vi "GUI_Cameras_v1.3.1.vi"() -> ()   [LabVIEW 2013]
uses:
  <vilib>/vision/NI_Vision_Development_Module.lvlib
  <vilib>/Utility/miscctls.llb/LVRectTypeDef.ctl
panel:
  in  "resize":bool
  in  "Tab Control":T1(tab)
  out "Max Counts":dbl(slide) scale=0.0..256.0
  in  "triggerdelay":dbl
  in  "trigger":bool
  in  "save":bool
  in  "exposure":dbl=0.52 caption="Exposure"
  in  "gain":dbl
  in  "shotnumber":i32=354
  in  "LogArray":bool
  in  "ROI.OffsetY":dbl
  in  "ROI.OffsetX":dbl
  in  "ROI.Height":dbl
  in  "ROI.Width":dbl
  in  "localanalysis":bool
  in  "MaxGUIPixel":dbl
  out "Centroid":cluster{"X Centroid":sgl, "Y Centroid":sgl} {"Y Centroid" format="%.2f"; "X Centroid" format="%.2f"}
  out "Y Resolution":i32
  out "X Resolution":i32
  out "Mean Value":sgl format="%.2f"
  out "GUIBinning":dbl
  in  "size":dbl=20.0
  in  "Target.Y":dbl
  in  "Target.X":dbl
  in  "draw Xhair":bool
  out "Mean Value 2":sgl(graph)
  out "histogram":T2(graph)
  out "lineout":cluster{"x0":sgl, "dx":sgl, "Pixels Line":sgl[]}(graph)
  out "MaxCounts":dbl
  in  "FWHMx":dbl
  in  "FWHMy":dbl
  out "MeanCounts":dbl
  out "FWHMx (um)":dbl
  out "FWHMy (um)":dbl
  in  "SpatialCalibration":dbl
  in  "Analysis":bool
  out "analysis error":errorcluster
  out "top":i16
  out "left":i16
  out "Zoom changed":bool
  out "Zoom old":cluster{"X":sgl, "Y":sgl}
  out "ratio(h)":bool=TRUE
  out "fixsize":bool
  out "Change Ratio":cluster{"X":sgl, "Y":sgl}={"X"=1.6671598, "Y"=0.6151203}
  out "old Panel Bounds":T3={"Left"=105, "Top"=80, "Right"=781, "Bottom"=662}
  out "error (h)":bool
  in  "Main Tap":enum32{"IMAQ", "Network", "Internal", "Array"}(tab)
  out "Image (IMAQ)":T4(plugin-control)
  out "local Port":u16=65401
  out "Remote Host":string="192.168.10.157"
  out "port or service name":u16=65400
  in  "timeout ms (slow resp)":i32=500
  in  "reset":bool
  out "All Devices (h)":string[](array[string])
  out "centroidy":dbl
  out "fast ID (h)":refnum<k16>
  out "slow ID (h)":refnum<k16>
  out "error out":errorcluster
  out "connections (hidden)":variant[](array[variant])=[variant(refnum<k16> refnum), variant(refnum<k16> refnum)]
  in  "time to wait (main loop)":i32=200
  in  "time to wait (TCP)":i32=10
  out "Data String":string="exposure,0.520000\r\ntrigger,off\r\nsave,off\r\ngain,0.000000\r\n"
  in  "send":bool
  in  "localsavingpath":path
  out "centroidy":dbl
  out "Image (array)":dbl[][](graph)
  out "Device Name (h)":string="FakeCam1"
  out "stop":bool
  out "error message":string
  out "image connection":bool
  out "data connection ok":bool
  # "Trigger"
  # "Save"
  # "Data"
  # "Image"
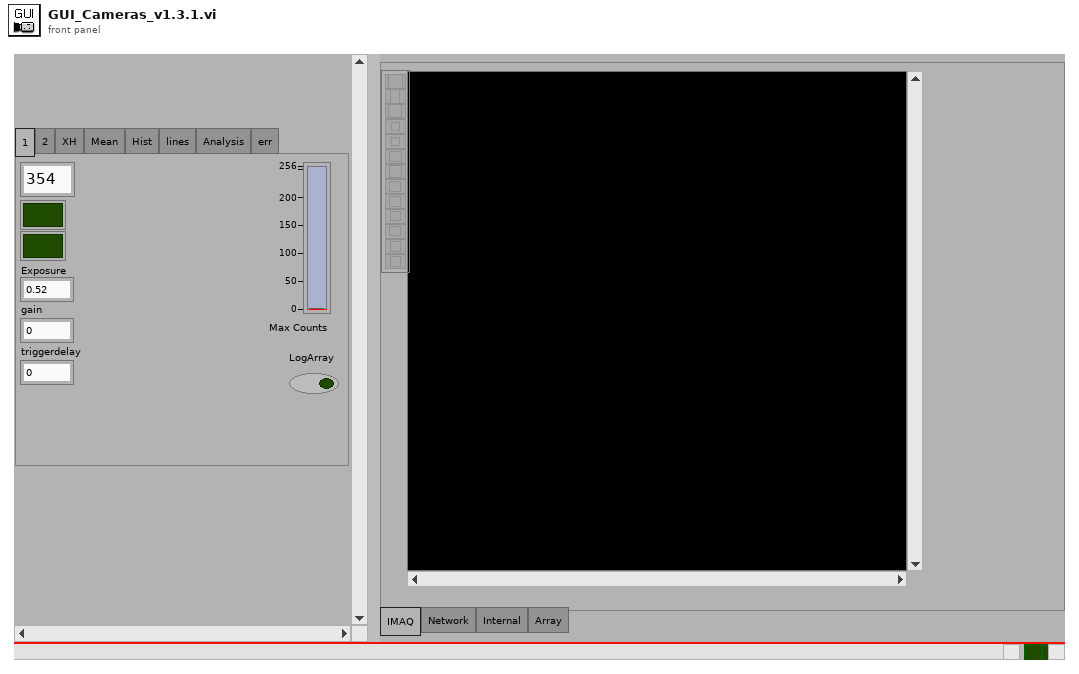
[diagram p1: front panel]
types:
  T1 = enum32{"1", "2", "XH", "Mean", "Hist", "lines", "Analysis", "err"}
  T2 = cluster{"Starting Value":sgl, "Incremental Value":sgl, "Histogram":u32[]}
  T3 = typedef "LVRectTypeDef.ctl" = cluster{"Left":i16, "Top":i16, "Right":i16, "Bottom":i16}
  T4 = typedef "IMAQ Image.ctl" = refnum<image>
  T5 = enum16{"Grayscale", "Binary", "Gradient", "Rainbow", "Temperature", "User Defined"}
  T6 = cluster{"Left":i32, "Top":i32, "Right":i32, "Bottom":i32}
  T7 = typedef "Image Type" = u32
  T8 = cluster{"Global Rectangle":i32[], "Contours":cluster{"Contour Type":u32, "ROI Type":u32, "Points":i32[]}[]}
  T9 = typedef "EventTypDef.ctl" = refnum<user-event>
  T10 = typedef "IMAQ Line" = cluster{"Start X":i32, "Start Y":i32, "End X":i32, "End Y":i32}
  T11 = typedef "LVBoundsTypeDef.ctl" = cluster{"Width":u32, "Height":u32}
  T12 = typedef "ROI Descriptor" = cluster{"Global Rectangle":i32[], "Contours":cluster{"ID":enum32{"External", "Internal"}, "Type":u32, "Coordinates":i32[]}[]}
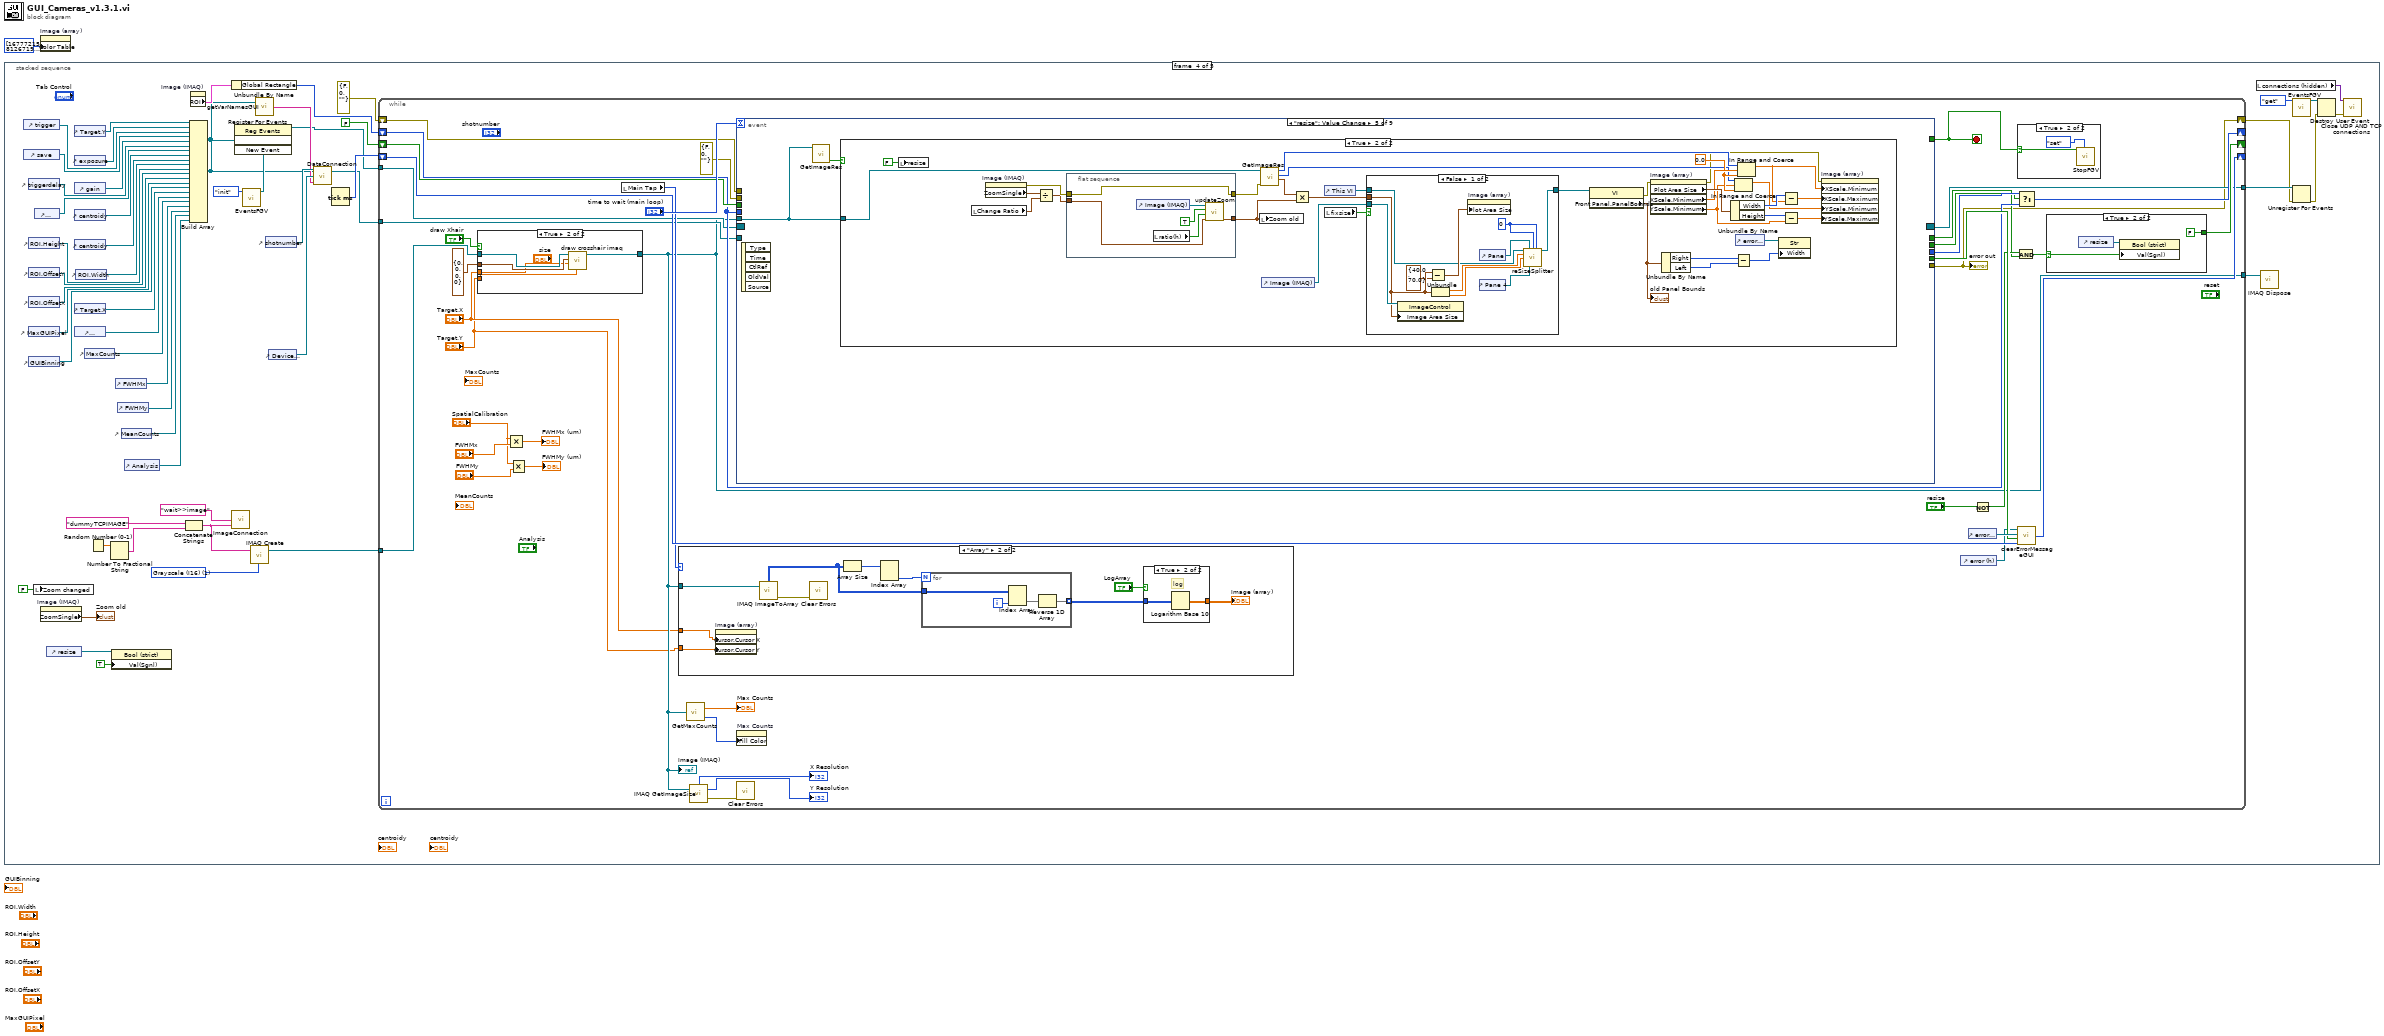
[diagram p0: block diagram]
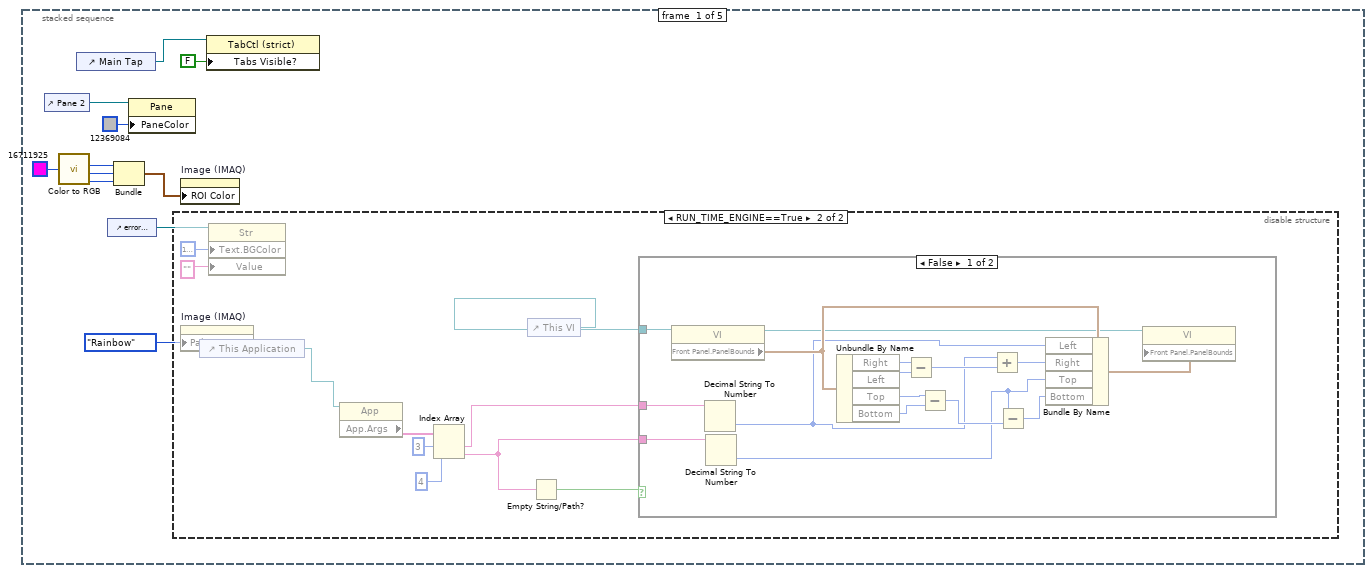
[diagram p2: hidden frame]
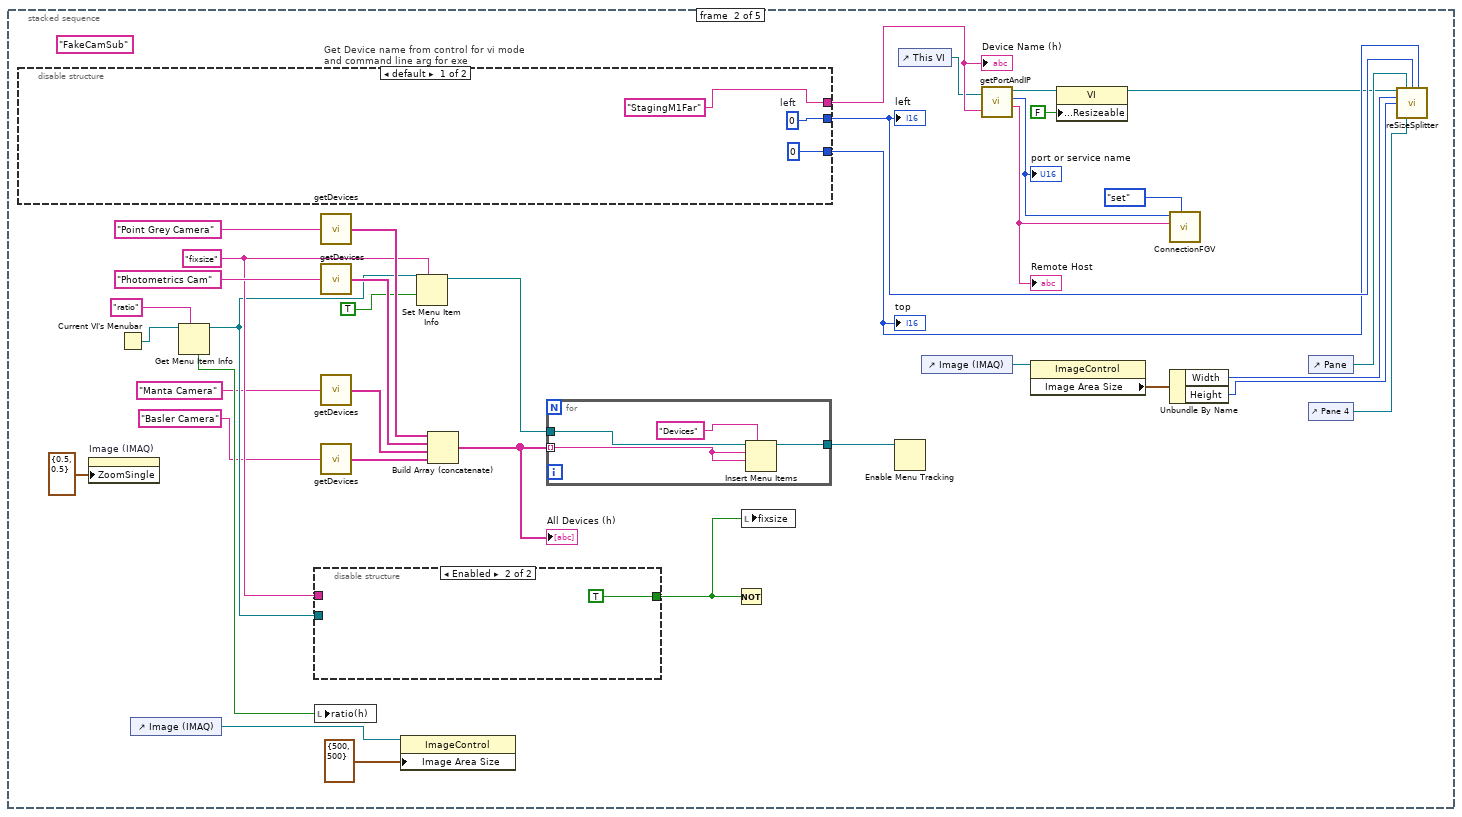
[diagram p5: hidden frame]
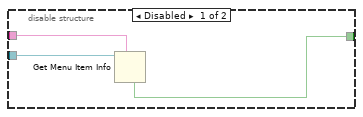
[diagram p6: hidden frame]
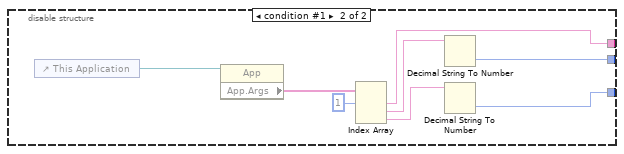
[diagram p7: hidden frame]
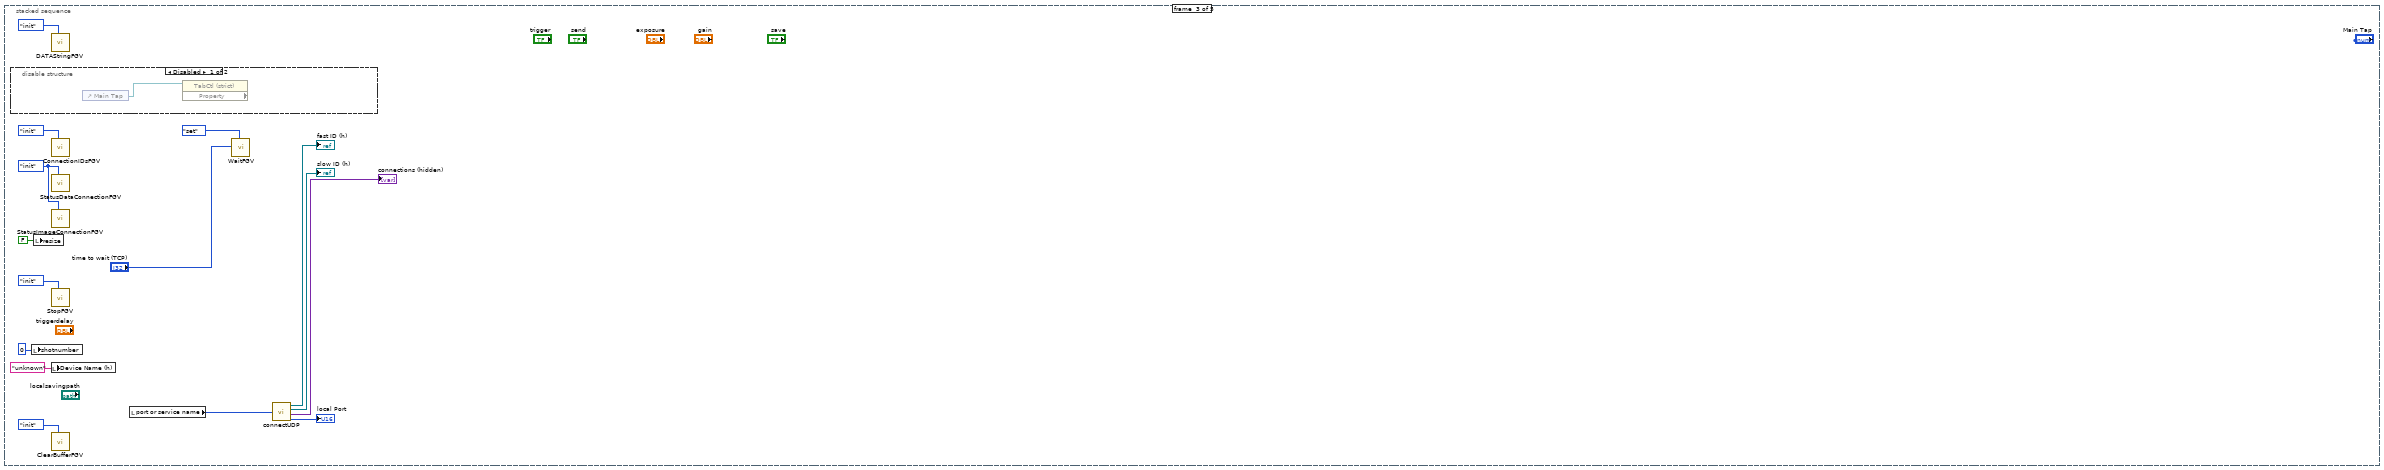
[diagram p8: hidden frame]
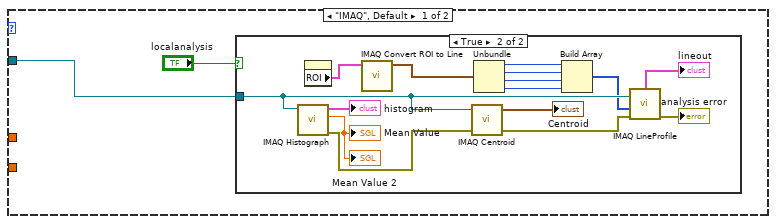
[diagram p13: hidden frame]
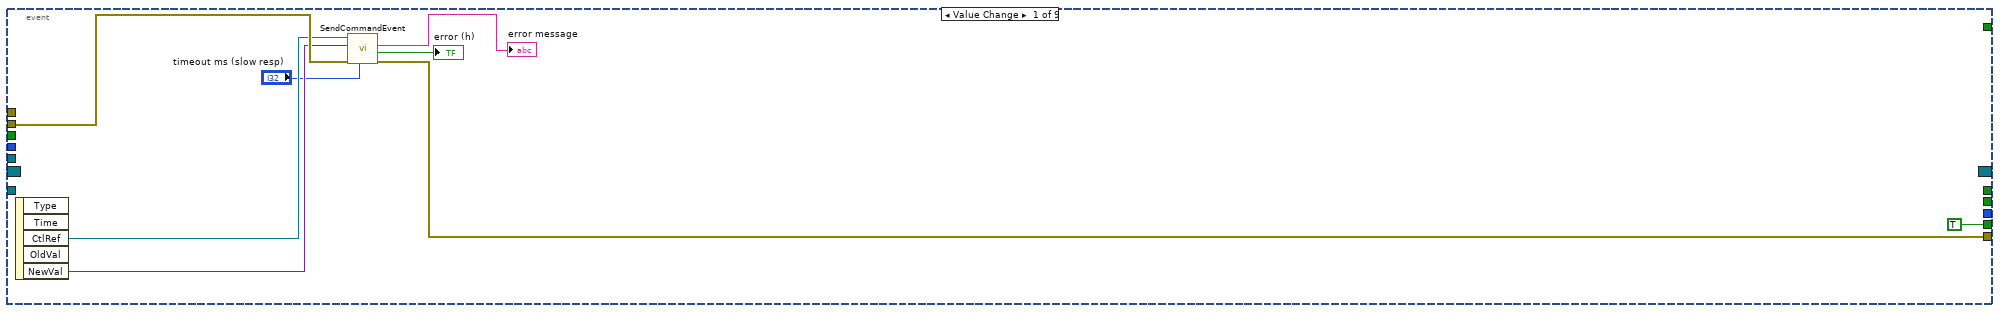
[diagram p16: hidden frame]
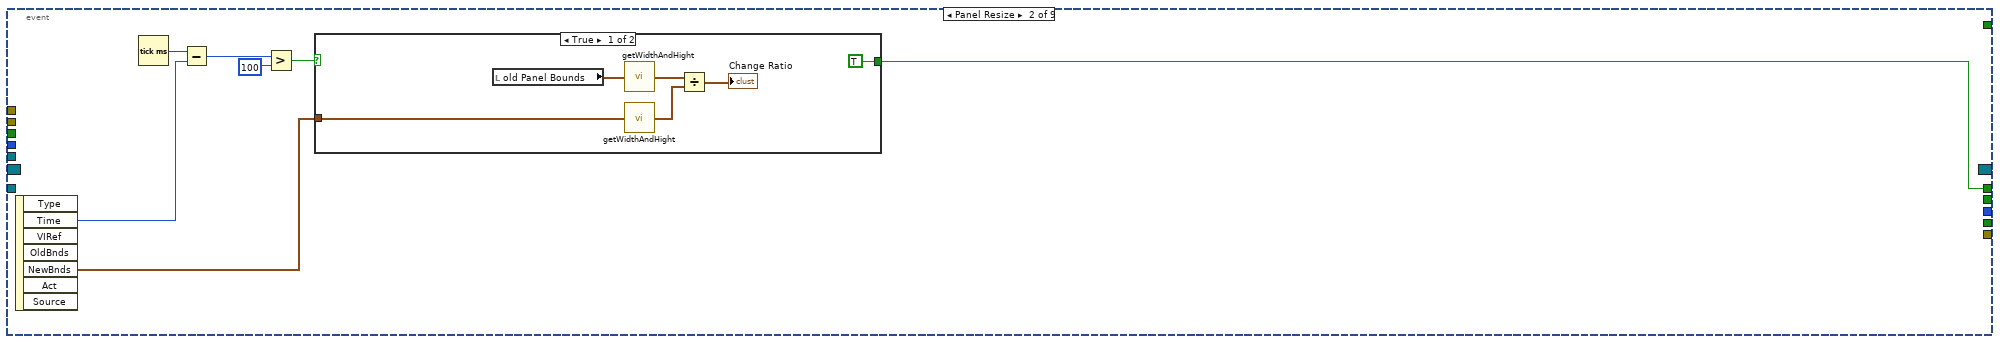
[diagram p17: hidden frame]
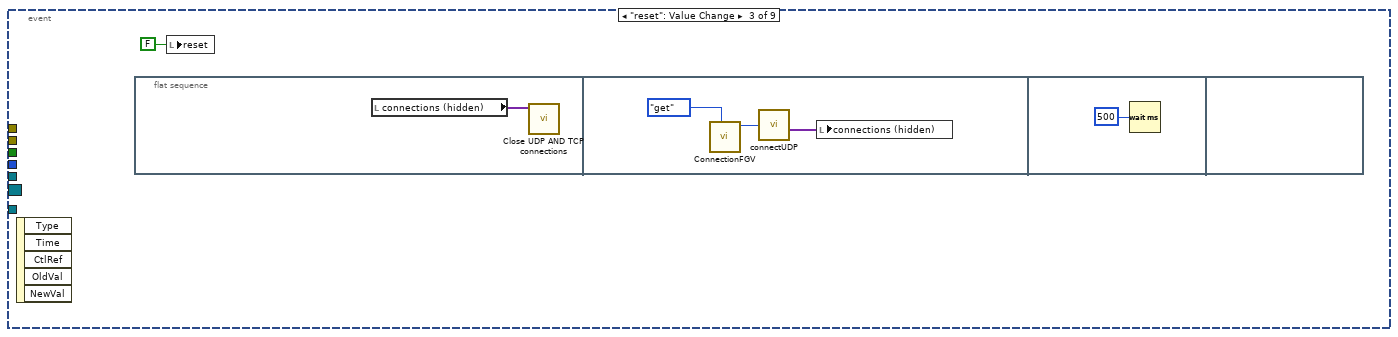
[diagram p19: hidden frame]
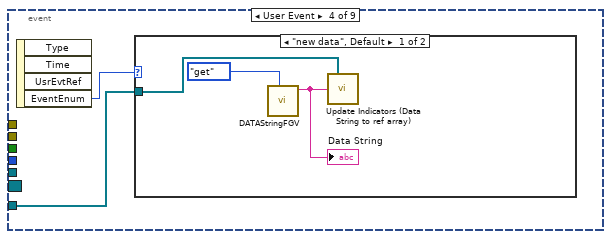
[diagram p20: hidden frame]
diagram:
  n1 = stacked-sequence {
    frame #0 {
      n2 = control-ref of="Pane 2"() -> (w9:refnum<vi>)
      n3 = call <vilib>:"Color to RGB.vi"("Color"=u32 16711925) -> ("R"=w5:u8, "G"=w4:u8, "B"=w3:u8)  [unwired: 1 out]
      n4 = control-ref of="Main Tap"() -> (w14:refnum<vi>)
      n5 = control-ref of="error message"() -> (w11:refnum<vi>)
      n6 = Bundle("R"=w5, "G"=w4, "B"=w3) -> (w2:cluster{"R":u8, "G":u8, "B":u8})  [unwired: 1 in]
      n7 = property class="Pane"(reference=w9, "PaneColor"=u32 12369084) -> ()  [unwired: 1 in, 2 out]
      n8 = disable-structure shown="RUN_TIME_ENGINE==True" {
        frame condition #0 (active) {
        }
        frame condition #1 {
          n9 = control-ref of="This Application"() -> (w15:refnum<vi>)
          n10 = property class="App"(reference=w15) -> ("App.Args"=w22:string[])  [unwired: 1 in, 2 out]
          n11 = Index Array(array=w22, index #1=3 ("index"), index #2=4 ("index")) -> (element #1=w19:string, element #2=w18:string)
          n12 = control-ref of="This VI"() -> (w16:refnum<vi>)
          n13 = Empty String/Path?(string/path=w18) -> (empty?=w17:bool)
          n14 = case shown="False" w17 {
            tunnel: w19 -> [w38 _]
            tunnel: w16 -> [w24 _]
            tunnel: w18 -> [w23 _]
            frame False {
              n15 = property class="VI"(reference=w24) -> (reference out=w28:refnum<vi>, "Front Panel.PanelBounds"=w33:T3)  [unwired: 1 in, 1 out]
              n16 = Decimal String To Number(string=w38) -> (number=w26:i32)  [unwired: 2 in, 1 out]
              n17 = Decimal String To Number(string=w23) -> (number=w25:i32)  [unwired: 2 in, 1 out]
              n18 = Unbundle By Name(w33) -> ("Right"=w29:i16, "Left"=w30:i16, "Top"=w31:i16, "Bottom"=w32:i16)
              n19 = Subtract(x=w29, y=w30) -> (x-y=w34:i16)
              n20 = Subtract(x=w31, y=w32) -> (x-y=w36:i16)
              n21 = Add(x=w26, y=w34) -> (x+y=w35:i32)
              n22 = Subtract(x=w25, y=w36) -> (x-y=w37:i32)
              n23 = Bundle By Name(cluster=w33, "Left"=w26, "Right"=w35, "Top"=w25, "Bottom"=w37) -> (w27:T3)
              n24 = property class="VI"(reference=w28, "Front Panel.PanelBounds"=w27) -> ()  [unwired: 1 in, 2 out]
            }
            frame True {
            }
          }
        }
      }
      n25 = property on="Image (IMAQ)" class="ImageControl"("ROI Color"=w2) -> ()  [unwired: 2 in, 2 out]
      n26 = property on="Image (IMAQ)" class="ImageControl"("Palette Type"=T5."Rainbow" ("Palette:Palette Type")) -> ()  [unwired: 2 in, 2 out]
      n27 = property class="TabCtl (strict)"(reference=w14, "Tabs Visible?"=FALSE) -> ()  [unwired: 1 in, 2 out]
      n28 = property class="Str"(reference=w11, "Text.BGColor"=u32 16777238, "Value"="") -> ()  [unwired: 1 in, 2 out]
    }
    frame #1 {
      (unwired) "FakeCamSub" ("Device Class")
      w46 = "fixsize" ("item tag")
      n29 = disable-structure "Get Device name from control for vi mode\nand command line arg for exe" shown="default" {
        disable-tunnel: ["StagingM1Far" ("Device Name for vi mode") w91] -> w61
        disable-tunnel: [w85 w88] -> w66
        disable-tunnel: [i16 0 ("left") w87] -> w65
        frame condition #0 (active) {
          w85 = i16 0  # left
        }
        frame condition #1 {
          n30 = control-ref of="This Application"() -> (w94:refnum<vi>)
          n31 = property class="App"(reference=w94) -> ("App.Args"=w93:string[])  [unwired: 1 in, 2 out]
          n32 = Index Array(array=w93, index #1=1 ("index")) -> (element #1=w91:string, element #2=w90:string, element #3=w89:string)  [unwired: 2 in]
          n33 = Decimal String To Number(string=w90) -> (number=w88:i32)  [unwired: 2 in, 1 out]
          n34 = Decimal String To Number(string=w89) -> (number=w87:i32)  [unwired: 2 in, 1 out]
        }
      }
      "Device Name (h)" <- w61
      "left" <- w66
      "top" <- w65
      n35 = property on="Image (IMAQ)" class="ImageControl"("ZoomSingle"=cluster{"X":sgl, "Y":sgl} {"X"=0.5, "Y"=0.5} ("ZoomSingle:All Elements")) -> ()  [unwired: 2 in, 2 out]
      n36 = Current VI's Menubar() -> (w68:refnum<k9>)
      n37 = control-ref of="Image (IMAQ)"() -> (w49:refnum<vi>)
      n38 = Get Menu Item Info(7:"ratio" ("item tag"), 11:w68) -> (3:w45:refnum<k9>, 4:w67:bool)  [unwired: 1 in, 5 out]
      n39 = disable-structure shown="Enabled" {
        disable-tunnel: [w78 TRUE] -> w64
        disable-tunnel: w46 -> [w77 _]
        disable-tunnel: w45 -> [w76 _]
        frame Disabled {
          n40 = Get Menu Item Info(7:w77, 11:w76) -> (4:w78:bool)  [unwired: 1 in, 6 out]
        }
        frame Enabled {
        }
      }
      n41 = local write "ratio(h)"(w67) -> ()
      n42 = call "getDevices.vi"("Device Class"="Point Grey Camera") -> ("All Devices"=w52:string[])
      n43 = call "getDevices.vi"("Device Class"="Photometrics Cam") -> ("All Devices"=w51:string[])
      n44 = call "getDevices.vi"("Device Class"="Manta Camera") -> ("All Devices"=w41:string[])
      n45 = call "getDevices.vi"("Device Class"="Basler Camera") -> ("All Devices"=w39:string[])
      n46 = property class="ImageControl"(reference=w49, "Image Area Size"=cluster{"Width":u32, "Height":u32} {"Width"=500, "Height"=500} ("Image Area:Size:All Elements")) -> ()  [unwired: 1 in, 2 out]
      n47 = Set Menu Item Info(7:w46, 9:TRUE ("enabled"), 11:w45) -> (3:w44:refnum<k9>)  [unwired: 4 in, 1 out]
      n48 = Build Array (concatenate)(w52, w51, w41, w39) -> (w50:string[])
      "All Devices (h)" <- w50
      n49 = for {
        tunnel: w44 -> [w83]
        tunnel: [w82] -> w62
        tunnel: w50 -> [w80] mode=indexing
        n50 = Insert Menu Items(5:"Devices" ("menu tag"), 7:w80, 8:w80, 9:w83) -> (3:w82:refnum<k9>)  [unwired: 2 in, 2 out]
      }
      n51 = Not(x=w64) -> ()  [unwired: 1 out]
      n52 = local write "fixsize"(w64) -> ()
      n53 = Enable Menu Tracking(4:w62) -> ()  [unwired: 2 in, 2 out]
      n54 = control-ref of="This VI"() -> (w60:refnum<vi>)
      n55 = control-ref of="Image (IMAQ)"() -> (w75:refnum<vi>)
      n56 = call "getPortAndIP.vi"("This Vi"=w60, "Device Name"=w61) -> ("reference out"=w59:refnum<vi>, "port or service name"=w56:u16, "Remote Host"=w55:string)  [unwired: 1 in]
      "port or service name" <- w56
      "Remote Host" <- w55
      n57 = property class="ImageControl"(reference=w75) -> ("Image Area Size"=w74:cluster{"Width":u32, "Height":u32})  [unwired: 1 in, 2 out]
      n58 = property class="VI"(reference=w59, "Front Panel.Resizeable"=FALSE ("Front Panel Window:Resizable")) -> (reference out=w58:refnum<vi>)  [unwired: 1 in, 1 out]
      n59 = call "ConnectionFGV.vi"("command"=enum16{"get", "set", "init"}."set", "Remote Host in"=w55, "port or service name in"=w56) -> ()  [unwired: 7 in, 2 out]
      n60 = Unbundle By Name(w74) -> ("Width"=w73:u32, "Height"=w72:u32)
      n61 = control-ref of="Pane"() -> (w71:refnum<vi>)
      n62 = control-ref of="Pane 4"() -> (w63:refnum<vi>)
      n63 = call "reSizeSplitter.vi"("this vi"=w58, "pane"=w71, "left"=w66, "top"=w65, "Width"=w73, "Height"=w72, "pane2"=w63) -> ()  [unwired: 8 in, 1 out]
    }
    frame #2 {
      w105 = enum16{"get", "set", "init"}."init" ("Command")
      n64 = disable-structure shown="Disabled" {
        frame Disabled {
          n65 = control-ref of="Main Tap"() -> (w110:refnum<vi>)
          n66 = property class="TabCtl (strict)" props=[](reference=w110) -> ()  [unwired: 1 in, 3 out]
        }
        frame Enabled {
        }
      }
      n67 = local write "shotnumber"(0 ("shotnumber")) -> ()
      n68 = local write "resize"(FALSE ("resize")) -> ()
      n69 = call "DATAStringFGV.vi"("Command"=enum16{"get", "set", "init"}."init") -> ()  [unwired: 9 in, 2 out]
      n70 = call "ConnectionIDsFGV.vi"("Command"=enum16{"add", "get", "init"}."init") -> ()  [unwired: 10 in, 1 out]
      n71 = call "StatusDataConnectionFGV.vi"("Command"=w105) -> ()  [unwired: 10 in, 1 out]
      n72 = call "StatusImageConnectionFGV.vi"("Command"=w105) -> ()  [unwired: 10 in, 1 out]
      n73 = call "StopFGV.vi"("Command"=enum16{"set", "get", "init"}."init") -> ()  [unwired: 9 in, 2 out]
      n74 = local write "Device Name (h)"("unknown" ("Device Name")) -> ()
      n75 = call "ClearBufferFGV.vi"("Command"=enum16{"set", "get", "init"}."init") -> ()  [unwired: 10 in, 1 out]
      n76 = local read "port or service name"() -> (w107:u16)
      n77 = call "WaitFGV.vi"("Command"=enum16{"get", "set", "init"}."set", "milliseconds to wait"="time to wait (TCP)") -> ()  [unwired: 9 in, 1 out]
      n78 = call "connectUDP.vi"("port or service name NOT USED"=w107) -> ("fast ID (h)"=→"fast ID (h)":refnum<k16>, "slow ID (h)"=→"slow ID (h)":refnum<k16>, "connections (hidden)"=→"connections (hidden)":variant[], "local Port"=→"local Port":u16)
    }
    frame #3 {
      w161 = T7 1 items=["Grayscale (U8)", "Grayscale (I16)", "Grayscale (SGL)", "Complex (CSG)", "RGB (U32)", "HSL (U32)", "RGB (U64)", "Grayscale (U16)"] ("Image Type")
      n79 = control-ref of="trigger"() -> (w153:refnum<vi>)
      n80 = control-ref of="save"() -> (w151:refnum<vi>)
      n81 = control-ref of="triggerdelay"() -> (w149:refnum<vi>)
      n82 = control-ref of="ROI.OffsetY"() -> (w122:refnum<vi>)
      n83 = control-ref of="ROI.OffsetX"() -> (w121:refnum<vi>)
      n84 = control-ref of="MaxGUIPixel"() -> (w120:refnum<vi>)
      n85 = control-ref of="ROI.Height"() -> (w123:refnum<vi>)
      n86 = control-ref of="GUIBinning"() -> (w119:refnum<vi>)
      n87 = local write "Zoom changed"(FALSE ("Zoom changed")) -> ()
      n88 = control-ref of="localsavingpath"() -> (w145:refnum<vi>)
      n89 = property on="Image (IMAQ)" class="ImageControl"() -> ("ZoomSingle"=→"Zoom old":cluster{"X":sgl, "Y":sgl})  [unwired: 2 in, 2 out]
      n90 = control-ref of="resize"() -> (w135:refnum<vi>)
      n91 = control-ref of="Target.Y"() -> (w117:refnum<vi>)
      n92 = control-ref of="exposure"() -> (w152:refnum<vi>)
      n93 = control-ref of="gain"() -> (w150:refnum<vi>)
      n94 = control-ref of="centroidy"() -> (w144:refnum<vi>)
      n95 = control-ref of="centroidy"() -> (w138:refnum<vi>)
      n96 = control-ref of="Target.X"() -> (w118:refnum<vi>)
      n97 = control-ref of="SpatialCalibration"() -> (w116:refnum<vi>)
      n98 = control-ref of="ROI.Width"() -> (w124:refnum<vi>)
      n99 = control-ref of="MaxCounts"() -> (w115:refnum<vi>)
      n100 = Random Number (0-1)() -> (number: 0 to 1=w159:dbl)
      n101 = Number To Fractional String(number=w159) -> (F-format string=w158:string)  [unwired: 3 in]
      n102 = property class="Bool (strict)"(reference=w135, "Val(Sgnl)"=TRUE ("Value (Signaling)")) -> ()  [unwired: 1 in, 2 out]
      n103 = control-ref of="FWHMx"() -> (w114:refnum<vi>)
      n104 = control-ref of="FWHMy"() -> (w113:refnum<vi>)
      n105 = control-ref of="MeanCounts"() -> (w112:refnum<vi>)
      n106 = control-ref of="Analysis"() -> (w111:refnum<vi>)
      n107 = Concatenate Strings("dummyTCPIMAGE" ("Image Name"), w158) -> (w156:string)
      n108 = Build Array(w117, w152, w153, w151, w150, w149, w145, w144, w138, w124, w123, w122, w121, w120, w119, w118, w116, w115, w114, w113, w112, w111) -> (w132:refnum<vi>[])
      n109 = property on="Image (IMAQ)" class="ImageControl"() -> ("ROI"=w143:T8)  [unwired: 2 in, 2 out]
      n110 = Unbundle By Name(w143) -> ("Global Rectangle"=w142:i32[])
      n111 = call "ImageConnection.vi"("Image Name"=w156, "Image Subscriber list"="wait>>image") -> ()  [unwired: 2 in]
      n112 = call "EventsFGV.vi"("Command"=enum16{"get", "init"}."init") -> ("New Event"=w133:T9)  [unwired: 9 in, 1 out]
      n113 = register-events(w132, w133) -> (reference out=w131:refnum<event-registration>)  [unwired: 2 in, 1 out]
      n114 = call "IMAQ Create"("Image Name"=w156, "Image Type"=w161) -> ("New Image"=w160:T4)  [unwired: 3 in, 1 out]
      n115 = call "getVarNamesGUI.vi"("Array"=w132) -> ("String"=w137:string)  [unwired: 1 in]
      n116 = control-ref of="shotnumber"() -> (w140:refnum<vi>)
      n117 = control-ref of="Device Name (h)"() -> (w139:refnum<vi>)
      n118 = call "DataConnection.vi"("Subscriber list"=w137, "Device Name (h)"=w139, "shotnumber"=w140) -> ()
      n119 = Tick Count (ms)() -> (millisecond timer value=w146:u32)
      n120 = while {
        shift-right: [w178] -> w128
        shift-left: errorcluster {"status"=FALSE, "code"=0, "source"=""} ("error out") -> [w201]
        tunnel: w160 -> [w174]
        tunnel: [w173] -> w162
        tunnel: w132 -> [w185]
        shift-right: [w184] -> _
        shift-left: FALSE -> [w200]
        shift-right: [w199] -> _
        shift-left: w146 -> [w198]
        shift-right: [w193] -> _
        shift-left: w142 -> [w192]
        tunnel: w131 -> [w186]
        tunnel: [w179] -> w130
        stop <- w187 stop-if-true
        n121 = case shown="True" "draw Xhair" {
          tunnel: "Target.Y" -> [_ w205]
          tunnel: "Target.X" -> [_ w206]
          tunnel: w174 -> [w204 w209]
          tunnel: [w204 w207] -> w173
          tunnel: T6 {"Left"=0, "Top"=0, "Right"=0, "Bottom"=0} ("Bounding Rectangle") -> [_ w208]
          frame False {
          }
          frame True {
            n122 = call "draw crosshair imaq.vi"(6:w205, "Crosshair"=w206, "Bounding Rectangle"=w208, "image in"=w209) -> ("image out"=w207:T4)  [unwired: 6 in, 1 out]
          }
        }
        "Image (IMAQ)" <- w173
        n123 = Multiply(x="SpatialCalibration", y="FWHMx") -> (x*y=→"FWHMx (um)":dbl)
        n124 = Multiply(x="SpatialCalibration", y="FWHMy") -> (x*y=→"FWHMy (um)":dbl)
        n125 = local read "Main Tap"() -> (w195:enum32{"IMAQ", "Network", "Internal", "Array"})
        n126 = case shown="\"Array\"" w195 {
          tunnel: w173 -> [w217 w242]
          tunnel: "Target.X" -> [_ w234]
          tunnel: "Target.Y" -> [_ w233]
          frame "IMAQ", Default {
            n127 = case shown="True" "localanalysis" {
              tunnel: w217 -> [_ w228]
              frame False {
              }
              frame True {
                n128 = call "IMAQ Histograph"("Image"=w228) -> ("error out"=w230:errorcluster, "Mean Value"=→"Mean Value" →"Mean Value 2":sgl, "Histogram Graph"=→"histogram":T2)  [unwired: 7 in, 1 out]
                n129 = property on="Image (IMAQ)" class="ImageControl"() -> ("ROI"=w224:T8)  [unwired: 2 in, 2 out]
                n130 = call "IMAQ Convert ROI to Line"("ROI Descriptor"=w224) -> ("Line"=w223:T10)  [unwired: 8 in, 1 out]
                n131 = call "IMAQ Centroid"("error in (no error)"=w230, "Image"=w228) -> ("error out"=w227:errorcluster, "Centroid"=→"Centroid":cluster{"X Centroid":sgl, "Y Centroid":sgl})  [unwired: 2 in]
                n132 = Unbundle(w223) -> ("Start X"=w222:i32, "Start Y"=w221:i32, "End X"=w220:i32, "End Y"=w219:i32)
                n133 = Build Array(w222, w221, w220, w219) -> (w218:i32[])
                n134 = call "IMAQ LineProfile"("error in (no error)"=w227, "Line Coordinates"=w218, "Image"=w228) -> ("error out"=→"analysis error":errorcluster, "Line Graph"=→"lineout":cluster{"x0":sgl, "dx":sgl, "Pixels Line":sgl[]})  [unwired: 2 in, 2 out]
              }
            }
          }
          frame "Array" {
            n135 = property on="Image (array)" class="IntGraph (strict)"("Cursor.Cursor X"=w234, "Cursor.Cursor Y"=w233) -> ()  [unwired: 2 in, 2 out]
            n136 = call "IMAQ ImageToArray"("Image"=w242) -> ("error out"=w241:errorcluster, "Image Pixels (U8)"=w239:u8[][])  [unwired: 3 in, 3 out]
            n137 = call <vilib>:"Clear Errors.vi"("error in (no error)"=w241) -> ()  [unwired: 6 in, 1 out]
            n138 = Array Size(array=w239) -> (size(s)=w240:i32[])
            n139 = Index Array(array=w240) -> (element #2=w238:i32)  [unwired: 2 in, 1 out]
            n140 = for {
              N: w238 -> [_]
              tunnel: w239 -> [w249]
              tunnel: [w247] -> w236 mode=indexing
              i -> [w246]
              n141 = Index Array(array=w249, index (col)=w246) -> (element=w248:u8[])  [unwired: 1 in]
              n142 = Reverse 1D Array(array=w248) -> (reversed array=w247:u8[])
            }
            n143 = case shown="True" "LogArray" {
              tunnel: w236 -> [w243 w245]
              tunnel: [w243 w244] -> w235
              frame False {
              }
              frame True {
                # "log"
                n144 = Logarithm Base 10(1:w245) -> (0:w244:dbl[][])
              }
            }
            "Image (array)" <- w235
          }
        }
        n145 = call "GetMaxCounts.vi"("New Image"=w173) -> ("Maximal Value"=→"Max Counts":sgl, "Color"=w189:u32)
        n146 = call "IMAQ GetImageSize"("Image"=w173) -> ("Y Resolution"=→"Y Resolution":i32, "X Resolution"=→"X Resolution":i32, "error out"=w175:errorcluster)  [unwired: 3 in]
        n147 = event shown="[4] \"resize\": Value Change" {
          selector: w186 -> [_ _ _ _ _ _ _ _ _]
          dyn-events: [_ _ _ _ _ _ _ _ _] -> w179
          timeout: "time to wait (main loop)" -> [_ _ _ _ _ _ _ _ _]
          tunnel: [w255 _ _ _ _ w340 _ _ _] -> w178
          tunnel: errorcluster {"status"=FALSE, "code"=0, "source"=""} ("error out") -> [w257 _ _ _ _ _ _ _ _]
          tunnel: w201 -> [_ _ _ _ _ w340 _ _ _]
          tunnel: [TRUE _ _ _ _ _ _ _ _] -> w196
          tunnel: [_ _ _ _ _ _ w344 _ _] -> w187
          tunnel: w200 -> [_ _ _ _ _ _ _ _ _]
          tunnel: [_ w263 _ _ _ _ _ _ _] -> w181
          tunnel: [_ _ _ _ _ _ _ _ w412] -> w194
          tunnel: w192 -> [_ _ _ _ _ _ _ _ w413]
          tunnel: [_ _ _ _ _ _ _ _ w411] -> w191
          tunnel: w173 -> [_ _ _ _ w287 _ _ _ w414]
          tunnel: w185 -> [_ _ _ w277 _ _ _ _ _]
          event Value Change {
            n148 = event-data() -> ("CtlRef"=w252:refnum<vi>, "NewVal"=w251:variant)  [unwired: 1 in, 3 out]
            n149 = call "SendCommandEvent.vi"("timeout ms (slow resp)"="timeout ms (slow resp)", "error out 2"=w257, "NewVal"=w251, "CtlRef"=w252) -> ("error out"=w255:errorcluster, "error (h)"=→"error (h)":bool, "error message"=→"error message":string)  [unwired: 4 in, 1 out]
          }
          event Panel Resize {
            n150 = event-data() -> ("Time"=w261:u32, "NewBnds"=w264:T3)  [unwired: 1 in, 5 out]
            n151 = Tick Count (ms)() -> (millisecond timer value=w262:u32)
            n152 = Subtract(x=w262, y=w261) -> (x-y=w260:u32)
            n153 = Greater?(x=w260, y=u32 100) -> (0:w258:bool)
            n154 = case shown="True" w258 {
              tunnel: w264 -> [w270 _]
              tunnel: [TRUE _] -> w263
              frame True {
                n155 = local read "old Panel Bounds"() -> (w269:T3)
                n156 = call "getWidthAndHight.vi"("OldBnds"=w269) -> ("output cluster"=w267:cluster{"X":sgl, "Y":sgl})
                n157 = call "getWidthAndHight.vi"("OldBnds"=w270) -> ("output cluster"=w266:cluster{"X":sgl, "Y":sgl})
                n158 = Divide(x=w267, y=w266) -> (x/y=→"Change Ratio":cluster{"X":sgl, "Y":sgl})
              }
              frame False {
              }
            }
          }
          event "reset": Value Change {
            n159 = event-data() -> ()  [unwired: 1 in, 5 out]
            n160 = flat-sequence {
              frame #0 {
                n161 = local read "connections (hidden)"() -> (w272:variant[])
                n162 = call "Close UDP AND TCP connections.vi"("appended array"=w272) -> ()  [unwired: 7 in]
              }
              frame #1 {
                n163 = call "ConnectionFGV.vi"("command"=enum16{"get", "set", "init"}."get") -> ("port or service name out"=w274:u16)  [unwired: 9 in, 1 out]
                n164 = call "connectUDP.vi"("port or service name NOT USED"=w274) -> ("connections (hidden)"=w273:variant[])  [unwired: 3 out]
                n165 = local write "connections (hidden)"(w273) -> ()
              }
              frame #2 {
                n166 = Wait (ms)(milliseconds to wait=u32 500) -> ()  [unwired: 1 out]
              }
              frame #3 {
              }
            }
            n167 = local write "reset"(FALSE ("reset")) -> ()
          }
          event User Event {
            n168 = event-data() -> ("EventEnum"=w278:enum16{"new data", "connection status update"})  [unwired: 1 in, 3 out]
            n169 = case shown="\"new data\", Default" w278 {
              tunnel: w277 -> [w280 _]
              frame "new data", Default {
                n170 = call "DATAStringFGV.vi"("Command"=enum16{"get", "set", "init"}."get") -> ("Data String out"=w279:string)  [unwired: 9 in, 1 out]
                "Data String" <- w279
                n171 = call "Update Indicators (Data String to ref array).vi"("Array"=w280, "Data String"=w279) -> ()  [unwired: 12 in, 2 out]
              }
              frame "connection status update" {
                n172 = call "StatusDataConnectionFGV.vi"("Command"=enum16{"get", "set", "init"}."get") -> ("Data Connection out"=→"image connection":bool)  [unwired: 10 in]
                n173 = call "StatusImageConnectionFGV.vi"("Command"=enum16{"get", "set", "init"}."get") -> ("Image Connection out"=→"data connection ok":bool)  [unwired: 10 in]
              }
            }
          }
          event "resize": Value Change {
            n174 = event-data() -> ()  [unwired: 1 in, 5 out]
            n175 = call "GetImageRes.vi"("Image"=w287) -> ("valid Image"=w286:bool)  [unwired: 6 in, 4 out]
            n176 = case shown="True" w286 {
              tunnel: w287 -> [_ w296]
              frame False {
                n177 = local write "resize"(FALSE ("resize")) -> ()
              }
              frame True {
                w304 = 0.0 ("lower limit")
                n178 = local write "resize"(FALSE ("resize")) -> ()
                n179 = local read "Change Ratio"() -> (w320:cluster{"X":sgl, "Y":sgl})
                n180 = property on="Image (IMAQ)" class="ImageControl"() -> (error out=w291:errorcluster, "ZoomSingle"=w321:cluster{"X":sgl, "Y":sgl})  [unwired: 2 in, 1 out]
                n181 = Divide(x=w321, y=w320) -> (x/y=w290:cluster{"X":sgl, "Y":sgl})
                n182 = flat-sequence {
                  tunnel: [w325] -> w289
                  tunnel: w290 -> [w323]
                  tunnel: [w322] -> w292
                  tunnel: w291 -> [w322]
                  frame #0 {
                    n183 = control-ref of="Image (IMAQ)"() -> (w327:refnum<vi>)
                    n184 = local read "ratio(h)"() -> (w326:bool)
                    n185 = call "updateZoom.vi"("Zoom old"=w323, "ratio(h)"=w326, "update Zoom"=TRUE, "imageRef"=w327) -> ("Zoom out"=w325:cluster{"X":sgl, "Y":sgl})  [unwired: 7 in]
                  }
                }
                n186 = local write "Zoom old"(w289) -> ()
                n187 = call "GetImageRes.vi"("error in (no error)"=w292, "Image"=w296) -> ("Image Area:Size:All Elements"=w297:cluster{"Width":u32, "Height":u32}, "Y Resolution"=w298:i32, "X Resolution"=w299:i32)  [unwired: 5 in, 2 out]
                n188 = control-ref of="Image (IMAQ)"() -> (w311:refnum<vi>)
                n189 = Multiply(x=w297, y=w289) -> (x*y=w319:cluster{sgl, sgl})
                n190 = control-ref of="This VI"() -> (w300:refnum<vi>)
                n191 = local read "fixsize"() -> (w312:bool)
                n192 = case shown="False" w312 {
                  tunnel: w319 -> [w332 _]
                  tunnel: w300 -> [w328 w339]
                  tunnel: [w335 w339] -> w317
                  tunnel: w311 -> [w334 _]
                  frame False {
                    w329 = i16 0 ("left")
                    n193 = property class="ImageControl"(reference=w334, "Image Area Size"=w332) -> ()  [unwired: 1 in, 2 out]
                    n194 = Subtract(x=w332, y=cluster{sgl, sgl} {40.0, 70.0}) -> (x-y=w331:cluster{sgl, sgl})
                    n195 = Unbundle(w332) -> (w337:sgl, w338:sgl)
                    n196 = property on="Image (array)" class="IntGraph (strict)"("Plot Area Size"=w331) -> ()  [unwired: 2 in, 2 out]
                    n197 = control-ref of="Pane"() -> (w336:refnum<vi>)
                    n198 = control-ref of="Pane 4"() -> (w333:refnum<vi>)
                    n199 = call "reSizeSplitter.vi"("this vi"=w328, "pane"=w336, "left"=w329, "top"=w329, "Width"=w337, "Height"=w338, "pane2"=w333) -> ("reference out"=w335:refnum<vi>)  [unwired: 8 in]
                  }
                  frame True {
                  }
                }
                n200 = property class="VI"(reference=w317) -> (error out=w295:errorcluster, "Front Panel.PanelBounds"=w316:T3)  [unwired: 1 in, 1 out]
                "old Panel Bounds" <- w316
                n201 = property on="Image (array)" class="IntGraph (strict)"(error in=w295) -> (error out=w294:errorcluster, "Plot Area Size"=w310:T11, "XScale.Minimum"=w305:dbl, "YScale.Minimum"=w303:dbl)  [unwired: 1 in, 1 out]
                n202 = Unbundle By Name(w316) -> ("Right"=w315:i16, "Left"=w314:i16)
                n203 = Unbundle By Name(w310) -> ("Width"=w309:u32, "Height"=w307:u32)
                n204 = In Range and Coerce(upper limit=w298, x=w303, lower limit=w304) -> (coerced(x)=w302:dbl)  [unwired: 1 out]
                n205 = Subtract(x=w315, y=w314) -> (x-y=w313:i16)
                n206 = control-ref of="error message"() -> (w318:refnum<vi>)
                n207 = In Range and Coerce(upper limit=w299, x=w305, lower limit=w304) -> (coerced(x)=w306:dbl)  [unwired: 1 out]
                n208 = property class="Str"(reference=w318, "Width"=w313) -> ()  [unwired: 1 in, 2 out]
                n209 = Subtract(x=w309, y=w306) -> (x-y=w308:dbl)
                n210 = Subtract(x=w307, y=w303) -> (x-y=w301:dbl)
                n211 = property on="Image (array)" class="IntGraph (strict)"(error in=w294, "XScale.Minimum"=w306, "XScale.Maximum"=w308, "YScale.Minimum"=w302, "YScale.Maximum"=w301) -> ()  [unwired: 1 in, 2 out]
              }
            }
          }
          event Timeout {
            n212 = event-data() -> ()  [unwired: 1 in, 2 out]
          }
          event Menu Selection (User) {
            n213 = event-data() -> ("MenuRef"=w341:refnum<k9>, "ItemTag"=w342:string)  [unwired: 1 in, 3 out]
            n214 = Equal?(x="Exit", y=w342) -> (x = y?=w344:bool)
            "stop" <- w344
            n215 = property on="Main Tap" class="TabCtl (strict)"() -> ("Value"=w346:enum32{"IMAQ", "Network", "Internal", "Array"})  [unwired: 2 in, 2 out]
            n216 = case shown="False" w344 {
              tunnel: w346 -> [w405 _]
              tunnel: w342 -> [w404 _]
              tunnel: [w401 errorcluster {"status"=FALSE, "code"=0, "source"=""} ("error out")] -> w343
              frame False {
                n217 = call <userlib>:"Set Enum String Value__ogtk.vi"("String Value"=w404, "Default Enum Value"=w405) -> ("error out"=w403:errorcluster, "Enum"=w407:variant)  [unwired: 8 in]
                n218 = Variant To Data(error in=w403, type=w405, Variant=w407) -> (data=w406:enum32{"IMAQ", "Network", "Internal", "Array"}, error out=w402:errorcluster)
                n219 = property on="Main Tap" class="TabCtl (strict)"(error in=w402, "Value"=w406) -> (error out=w401:errorcluster)  [unwired: 1 in, 1 out]
              }
              frame True {
              }
            }
            n220 = case shown="Error" w343 {
              tunnel: w341 -> [_ w350]
              tunnel: w342 -> [_ w354]
              tunnel: [_ w355] -> _
              frame No Error {
              }
              frame Error {
                n221 = local read "All Devices (h)"() -> (w352:string[])
                n222 = Search 1D Array(1D array=w352, element=w354) -> (index of element=w353:i32)  [unwired: 1 in]
                n223 = Get Menu Item Info(7:w354, 11:w350) -> (0:w351:errorcluster, 2:w357:string, 4:w358:bool)  [unwired: 1 in, 4 out]
                n224 = Not(x=w358) -> (.not. x?=w356:bool)
                n225 = Greater Or Equal To 0?(x=w353) -> (x >= 0?=w349:bool)
                n226 = case shown="True" w349 {
                  tunnel: w352 -> [_ w362]
                  tunnel: w351 -> [_ _]
                  tunnel: w350 -> [w359 w361]
                  tunnel: [w359 w360] -> w348
                  frame False {
                  }
                  frame True {
                    n227 = for {
                      tunnel: w362 -> [w366] mode=indexing
                      tunnel: w361 -> [w364]
                      tunnel: [w363] -> w360
                      n228 = Set Menu Item Info(6:FALSE ("checked"), 7:w366, 11:w364) -> (3:w363:refnum<k9>)  [unwired: 4 in, 1 out]
                    }
                  }
                }
                n229 = case shown="Default" w354 {
                  selector: w354 -> [_ w372 _ _ w393 _ _]
                  tunnel: w356 -> [w367 w370 w383 _ _ _ w398]
                  tunnel: [_ _ TRUE _ _ _ _] -> w355
                  tunnel: w349 -> [_ w373 _ _ _ _ _]
                  tunnel: [w367 w371 w383 _ _ _ w398] -> w347
                  frame "fixsize" {
                    n230 = Not(x=w367) -> (.not. x?=w368:bool)
                    n231 = control-ref of="This VI"() -> (w369:refnum<vi>)
                    n232 = property class="VI"(reference=w369, "Front Panel.Resizeable"=w368) -> ()  [unwired: 1 in, 2 out]
                    "fixsize" <- w367
                  }
                  frame Default {
                    n233 = case shown="True" w373 {
                      tunnel: w372 -> [_ w381]
                      tunnel: [_ w377] -> w371
                      tunnel: w370 -> [_ w377]
                      frame False {
                      }
                      frame True {
                        n234 = control-ref of="This VI"() -> (w380:refnum<vi>)
                        n235 = control-ref of="reset"() -> (w379:refnum<vi>)
                        n236 = call "getPortAndIP.vi"("This Vi"=w380, "Device Name"=w381) -> ("port or service name"=w375:u16, "Remote Host"=w374:string)  [unwired: 1 in, 1 out]
                        n237 = local write "port or service name"(w375) -> ()
                        n238 = local write "Remote Host"(w374) -> ()
                        n239 = property class="Bool (strict)"(reference=w379, "Val(Sgnl)"=TRUE ("Value (Signaling)")) -> ()  [unwired: 1 in, 2 out]
                        n240 = call "ConnectionFGV.vi"("command"=enum16{"get", "set", "init"}."set", "Remote Host in"=w374, "port or service name in"=w375) -> ()  [unwired: 7 in, 2 out]
                      }
                    }
                  }
                  frame "ratio" {
                    n241 = property on="Image (IMAQ)" class="ImageControl"() -> ("ZoomSingle"=w382:cluster{"X":sgl, "Y":sgl})  [unwired: 2 in, 2 out]
                    n242 = local write "Zoom old"(w382) -> ()
                    "ratio(h)" <- w383
                  }
                  frame "Local Saving Path" {
                    n243 = control-ref of="localsavingpath"() -> (w385:refnum<vi>)
                    n244 = property class="Path"(reference=w385) -> (reference out=w388:refnum<vi>, "Value"=w389:path)  [unwired: 1 in, 1 out]
                    n245 = call "changePath.vi"("Local Saving in (h)"=w389) -> ("change (h)"=w387:bool, "Local Saving out (h)"=w386:path)  [unwired: 9 in]
                    n246 = case shown="True" w387 {
                      tunnel: w388 -> [_ w391]
                      tunnel: w386 -> [_ w390]
                      frame False {
                      }
                      frame True {
                        n247 = property class="Path"(reference=w391, "Val(Sgnl)"=w390) -> ()  [unwired: 1 in, 2 out]
                      }
                    }
                  }
                  frame "Binary", "Gradient", "Grayscale", "Rainbow", "Temperature" {
                    n248 = Scan From String(input string=w393, default 1=T5."Grayscale" ("Palette:Palette Type")) -> (output 1=w392:T5)  [unwired: 3 in, 3 out]
                    n249 = property on="Image (IMAQ)" class="ImageControl"("Palette Type"=w392) -> ()  [unwired: 2 in, 2 out]
                  }
                  frame "reset" {
                    n250 = control-ref of="reset"() -> (w396:refnum<vi>)
                    n251 = property class="Bool (strict)"(reference=w396, "Val(Sgnl)"=TRUE ("Value (Signaling)")) -> ()  [unwired: 1 in, 2 out]
                  }
                  frame "clear" {
                    n252 = control-ref of="reset"() -> (w400:refnum<vi>)
                    n253 = call "ClearBufferFGV.vi"("Command"=enum16{"set", "get", "init"}."set", "clear buffer"=w398) -> ()  [unwired: 9 in, 1 out]
                    n254 = property class="Bool (strict)"(reference=w400, "Val(Sgnl)"=TRUE ("Value (Signaling)")) -> ()  [unwired: 1 in, 2 out]
                  }
                }
                n255 = Set Menu Item Info(6:w347, 7:w354, 10:w357, 11:w348) -> ()  [unwired: 3 in, 2 out]
              }
            }
          }
          event "time to wait (TCP)": Value Change {
            n256 = event-data() -> ("NewVal"=w410:i32)  [unwired: 1 in, 4 out]
            n257 = call "WaitFGV.vi"("Command"=enum16{"get", "set", "init"}."set", "milliseconds to wait"=w410) -> ()  [unwired: 9 in, 1 out]
          }
          event "Image (IMAQ)": Mouse Up {
            n258 = event-data() -> ()  [unwired: 1 in, 5 out]
            n259 = disable-structure shown="Disabled" {
              disable-tunnel: w414 -> [w429 _]
              disable-tunnel: w413 -> [w427 _]
              disable-tunnel: [w426 _] -> w412
              disable-tunnel: [w420 _] -> w411
              frame Disabled {
                n260 = local read "Zoom old"() -> (w417:cluster{"X":sgl, "Y":sgl})
                n261 = property on="Image (IMAQ)" class="ImageControl"() -> ("ZoomSingle"=w416:cluster{"X":sgl, "Y":sgl})  [unwired: 2 in, 2 out]
                n262 = property on="Image (IMAQ)" class="ImageControl"() -> ("ROI"=w428:T8)  [unwired: 2 in, 2 out]
                n263 = Unbundle By Name(w428) -> ("Global Rectangle"=w426:i32[])
                n264 = Unbundle By Name(w416) -> ("X"=w418:sgl)
                n265 = Unbundle By Name(w417) -> ("X"=w419:sgl)
                n266 = Not Equal?(x=w427, y=w426) -> (x != y?=w430:bool[])
                n267 = Empty Array?(array=w426) -> (empty?=w425:bool)
                n268 = Not Equal?(x=w418, y=w419) -> (x != y?=w415:bool)
                "Zoom changed" <- w415
                n269 = Empty Array?(array=w427) -> (empty?=w423:bool)
                n270 = Or Array Elements(Boolean array=w430) -> (logical OR=w421:bool)
                n271 = Not(x=w425) -> (.not. x?=w424:bool)
                n272 = case shown="True" w415 {
                  tunnel: w416 -> [_ w433]
                  frame False {
                  }
                  frame True {
                    n273 = local write "Zoom old"(w433) -> ()
                  }
                }
                n274 = case shown="True" w415 {
                  selector: w415 -> [_ w431]
                  frame False {
                  }
                  frame True {
                    n275 = control-ref of="resize"() -> (w432:refnum<vi>)
                    n276 = property class="Bool (strict)"(reference=w432, "Val(Sgnl)"=w431) -> ()  [unwired: 1 in, 2 out]
                  }
                }
                n277 = And(x=w423, y=w424) -> (x .and. y?=w422:bool)
                n278 = Or(x=w421, y=w422) -> (x .or. y?=w420:bool)
                n279 = case shown="True" w420 {
                  tunnel: w429 -> [_ _]
                  tunnel: w428 -> [_ w435]
                  frame False {
                  }
                  frame True {
                    n280 = call "ROI thickener.vi"("ROI Descriptor in"=w435) -> ("ROI Descriptor out"=w434:T12)  [unwired: 1 in, 1 out]
                    n281 = property on="Image (IMAQ)" class="ImageControl"("ROI"=w434) -> ()  [unwired: 2 in, 2 out]
                  }
                }
              }
              frame Enabled {
              }
            }
          }
        }
        "error out" <- w178
        n282 = property on="Max Counts" class="Slide (strict)"("Fill Color"=w189) -> ()  [unwired: 2 in, 2 out]
        n283 = call <vilib>:"Clear Errors.vi"("error in (no error)"=w175) -> ()  [unwired: 6 in, 1 out]
        n284 = control-ref of="error (h)"() -> (w188:refnum<vi>)
        n285 = control-ref of="error message"() -> (w197:refnum<vi>)
        n286 = Not(x="resize") -> (.not. x?=w182:bool)
        n287 = And(x=w182, y=w181) -> (x .and. y?=w180:bool)
        n288 = case shown="True" w187 {
          selector: w187 -> [_ w214]
          frame False {
          }
          frame True {
            n289 = call "StopFGV.vi"("Command"=enum16{"set", "get", "init"}."set", "Stop"=w214) -> ()  [unwired: 8 in, 2 out]
          }
        }
        n290 = Select(t=w194, s=w191, f=w192) -> (s? t:f=w193:i32[])
        n291 = call "clearErrorMessageGUI.vi"("millisecond timer value"=w198, "Boolean"=w196, "error message"=w197, "reference"=w188) -> ("millisecond timer value 2"=w199:u32)
        n292 = case shown="True" w180 {
          selector: w180 -> [w210 w212]
          tunnel: [w210 FALSE] -> w184
          frame False {
          }
          frame True {
            n293 = control-ref of="resize"() -> (w213:refnum<vi>)
            n294 = property class="Bool (strict)"(reference=w213, "Val(Sgnl)"=w212) -> ()  [unwired: 1 in, 2 out]
          }
        }
      }
      n295 = local read "connections (hidden)"() -> (w155:variant[])
      n296 = call "IMAQ Dispose"("Image"=w162) -> ()  [unwired: 5 in, 1 out]
      n297 = call "EventsFGV.vi"("Command"=enum16{"get", "init"}."get") -> ("New Event"=w125:T9)  [unwired: 9 in, 1 out]
      n298 = Unregister For Events(event registration refnum=w130, error in=w128) -> (error out=w129:errorcluster)
      n299 = Destroy User Event(user event=w125, error in=w129) -> (error out=w127:errorcluster)
      n300 = call "Close UDP AND TCP connections.vi"("error in"=w127, "appended array"=w155) -> ()  [unwired: 6 in]
    }
    frame #4 {
      n301 = flat-sequence {
        frame #0 {
          n302 = Wait (ms)(milliseconds to wait=u32 0) -> ()  [unwired: 1 out]
        }
        frame #1 {
          n303 = local write "stop"(FALSE ("stop")) -> ()
        }
        frame #2 {
          n304 = control-ref of="This VI"() -> (w443:refnum<vi>)
          n305 = case shown="True" FALSE {
            tunnel: w443 -> [w444 w447]
            tunnel: [w444 w445] -> w442
            frame False {
            }
            frame True {
              n306 = property class="VI" props=["Front Panel.Open"](reference=w447) -> (reference out=w446:refnum<vi>)  [unwired: 1 in, 2 out]
              n307 = invoke class="VI" method="FP.Close"(reference=w446) -> (reference out=w445:refnum<vi>)  [unwired: 2 in, 2 out]
            }
          }
          n308 = Close Reference(reference=w442) -> ()  [unwired: 1 in, 1 out]
        }
      }
      n309 = control-ref of="Main  Control"() -> (w437:refnum<vi>)
      n310 = property class="TabCtl (strict)"(reference=w437, "Tab Location"=enum32{"Top", "Bottom", "Left", "Right"}."Bottom") -> ()  [unwired: 1 in, 2 out]
      n311 = property class="TabCtl (strict)"(reference=w437, "Tabs Visible?"=TRUE) -> ()  [unwired: 1 in, 2 out]
    }
  }
  n312 = property on="Image (array)" class="IntGraph (strict)"("Color Table"=u32[] [16777215, 8126719, 7864574, 7536895, 7274750, 6947071, 6684926, 6357247, 6095102, 5767423, 5505278, 5177599, 4915454, 4587775, 4325630, 3997951, 3735806, 3408127, 3145982, 2818303, 2556158, 2228479, 1966334, 1638655, 1376510, 1048831, 786686, 459007, 196862, 767, 1790, 3071, 4094, 5375, 6398, 7679, 8702, 9983, 11006, 12287, 13310, 14591, 15614, 16895, 17918, 19199, 20222, 21503, 22526, 23807, 24830, 26111, 27134, 28415, 29438, 30719, 31486, 33023, 33790, 35327, 36094, 37631, 38398, 39935, 40702, 42239, 43006, 44543, 45310, 46847, 47614, 49151, 49918, 51455, 52222, 53759, 54526, 56063, 56830, 58367, 59134, 60671, 61694, 62975, 63998, 65279, 65274, 65527, 65265, 65518, 65256, 65509, 65247, 65500, 65238, 65491, 65229, 65482, 65220, 65473, 65211, 65464, 65202, 65455, 65193, 65446, 65184, 65437, 65175, 65428, 65166, 65419, 65157, 65410, 65149, 65401, 65140, 65392, 65131, 65383, 65122, 65374, 65113, 65365, 65104, 65356, 65095, 65347, 65086, 65338, 65077, 65329, 65068, 65320, 65059, 65311, 65050, 65302, 65041, 65293, 65032, 65284, 130560, 392960, 720384, 982784, 1310208, 1572608, 1900032, 2162432, 2489856, 2752256, 3079680, 3342080, 3669504, 3931904, 4259328, 4521728, 4849152, 5111552, 5438976, 5701376, 6028800, 6291200, 6618624, 6881024, 7208448, 7470848, 7798272, 8126208, 8322560, 8716032, 8912384, 9305856, 9502208, 9895680, 10092032, 10485504, 10681856, 11075328, 11271680, 11665152, 11861504, 12254976, 12451328, 12844800, 13041152, 13434624, 13630976, 14024448, 14220800, 14614272, 14810624, 15204096, 15400448, 15793920, 15990272, 16383744, 16580096, 16776192, 16709376, 16773888, 16707072, 16771584, 16704768, 16769280, 16702464, 16766976, 16700160, 16764672, 16697856, 16762368, 16695552, 16760064, 16693248, 16757760, 16690944, 16755456, 16688640, 16753152, 16686336, 16750848, 16684032, 16748544, 16681728, 16746240, 16679680, 16743936, 16677376, 16741632, 16675072, 16739328, 16672768, 16737024, 16670464, 16734720, 16668160, 16732416, 16665856, 16730112, 16663552, 16727808, 16661248, 16725504, 16658944, 16723200, 16656640, 16720896, 16654336, 16718592, 16652032, 16716288, 16649728, 16713984, 16712960, 0] ("256 rainbow")) -> ()  [unwired: 2 in, 2 out]
